vi "Kill uService.vi"(8 "error in (no error)":errorcluster, 10 "uService":string, 11 "Guardian in":refnum<class "Guardian.lvclass">) -> (0 "error out":errorcluster, 3 "Guardian out":refnum<class "Guardian.lvclass">)   [LabVIEW 2026, in "TALOS.lvlib" / "Guardian.lvlib" / "Guardian.lvclass"]
uses:
  Guardian.lvclass
  Classes/uService List/uService List.lvclass/uService List.ctl
  Ancestor/Ancestor/Ancestor.lvclass/Ancestor.ctl
  Classes/uService List/Get Queue.vi
  Classes/uService List/Set Online Status.vi
  Support VIs/Generate Error.vi
  FGV/Error Memory/Get Error Description.vi
  Support VIs/Get PC name.vi
  Ancestor/Ancestor/Read ID.vi
  Support VIs/Get Class Name.vi
  <vilib>/Utility/error.llb/Clear Errors.vi
  FGV/Error Memory/Error Memory Core.vi
  <vilib>/AdvancedString/Delimited String to 1D String Array.vi
  <vilib>/AdvancedString/Delimited String to 1D String Array (string).vi
  Support VIs/Circus Root Path.vi
  FGV/Error Memory/Error Crt Lvl checker.vi
  FGV/Error Memory/Error Memory Core.vi/40c8088d-b597-4017-91af-faa98e00292e.vi
  FGV/Error Memory/Error Memory Core.vi/d4a3ab98-063c-4e44-b43d-fbdcfe6c2be2.vi
  Support VIs/Global Memory.vi
  <vilib>/Utility/LVClass/Get LV Class Name.vi
  Support VIs/Is in Packed Library.vi
  Support VIs/TALOS Root path.vi
  Support VIs/Read CSV worksheet.vi
  Support VIs/Global Constants.vi
  <vilib>/Utility/error.llb/General Error Handler.vi
  Support VIs/Error Log.vi
  builds/Actor Framework PPL/Actor Framework.lvlibp/1abvi3w/vi.lib/ActorFramework/Message Enqueuer/Message Enqueuer.lvclass
  Ancestor/Ancestor/Ancestor.lvclass
  <vilib>/Comparison/Equal/Equal Functor/Equal Functor.lvclass
  Classes/uService List/uService List.lvclass
  builds/Actor Framework PPL/Actor Framework.lvlibp/1abvi3w/vi.lib/ActorFramework/Stop Msg/Stop Msg.lvclass
  TALOS.lvlib
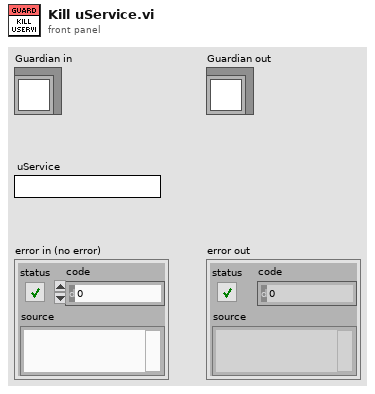
[diagram p1: front panel]
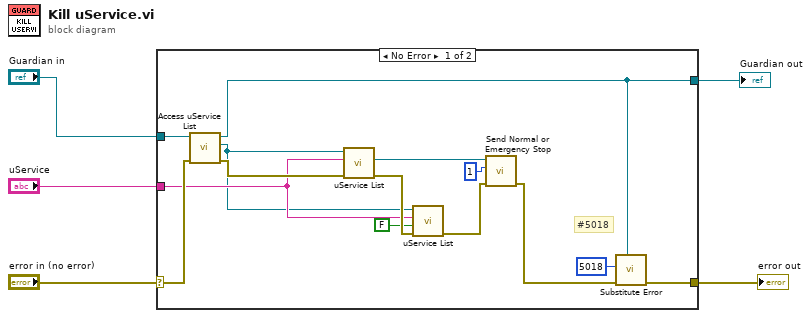
[diagram p0: block diagram]
diagram:
  n1 = case shown="No Error" "error in (no error)" {
    selector: "error in (no error)" -> [w16 w20]
    tunnel: [w8 w20] -> w5
    tunnel: "uService" -> [w15 _]
    tunnel: "Guardian in" -> [w14 w21]
    tunnel: [w7 w21] -> w1
    frame No Error {
      # "#5018"
      n2 = call-dynamic "Access uService List.vi"("error in (no error)"=w16, "Ancestor in"=w14) -> ("error out"=w17:errorcluster, "uService List out"=w13:refnum<class "uService List.lvclass">, "Ancestor out"=w7:refnum<class "Guardian.lvclass">)  [unwired: 7 in]
      n3 = call-poly "uService List.vi"("error in (no error)"=w17, "ID"=w15, "uService List in"=w13) -> ("error out"=w18:errorcluster, "uService Queue"=w12:refnum<class "Message Enqueuer.lvclass">)  [unwired: 6 in, 1 out]
      n4 = call-poly "uService List.vi"("error in (no error)"=w18, "Online"=FALSE, "ID"=w15, "uService List in"=w13) -> ("error out"=w19:errorcluster)  [unwired: 6 in, 1 out]
      n5 = call "Send Normal or Emergency Stop.vi"("error in (no error)"=w19, "final error code"=1, "Message Enqueuer"=w12) -> ("error out"=w9:errorcluster)  [unwired: 8 in]
      n6 = call "Substitute Error.vi"("LabVIEW Object"=w7, "error in (no error)"=w9, "Error Code"=5018) -> ("error out"=w8:errorcluster)  [unwired: 8 in]
    }
    frame Error {
    }
  }
  "error out" <- w5
  "Guardian out" <- w1
